vi "Parse DAC String Telemetry.vi"(10 "Variant":variant) -> (2 "DAC_RX_TLM":T1 {"DAC_1"."DATA" format="%04x"; "DAC_2"."DATA" format="%04x"; "DAC_3"."DATA" format="%04x"})   [LabVIEW 2019]
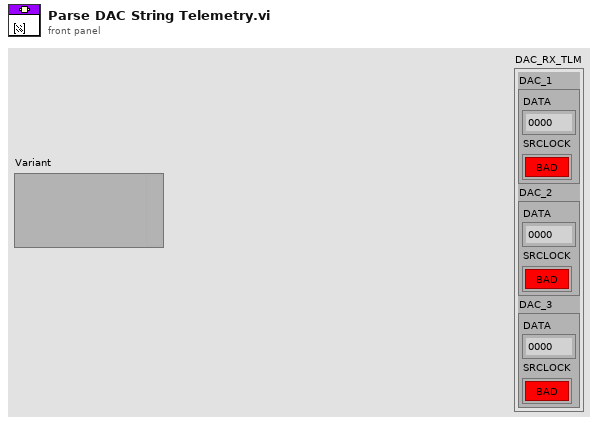
[diagram p1: front panel]
types:
  T1 = cluster{"DAC_1":cluster{"DATA":u16, "SRCLOCK":bool}, "DAC_2":cluster{"DATA":u16, "SRCLOCK":bool}, "DAC_3":cluster{"DATA":u16, "SRCLOCK":bool}}
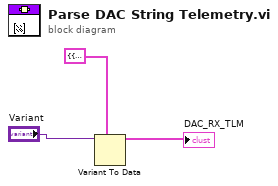
[diagram p0: block diagram]
diagram:
  n1 = Variant To Data(type=T1 {"DAC_1"={"DATA"=0, "SRCLOCK"=FALSE}, "DAC_2"={"DATA"=0, "SRCLOCK"=FALSE}, "DAC_3"={"DATA"=0, "SRCLOCK"=FALSE}}, Variant="Variant") -> (data=→"DAC_RX_TLM":T1)  [unwired: 1 in, 1 out]
